vi "create_batch-default.vi"(8 "error in (no error)":errorcluster, 9 "application_command":string, 10 "application_zip":string, 11 "target_directory":path) -> (0 "error out":errorcluster, 3 "batch_file":path)   [LabVIEW 2015, in "lv-builder-l3.lvlib"]
uses:
  lv-builder-l3.lvlib
  lv-build/lv-build.lvlib
panel:
  out "batch_file":string
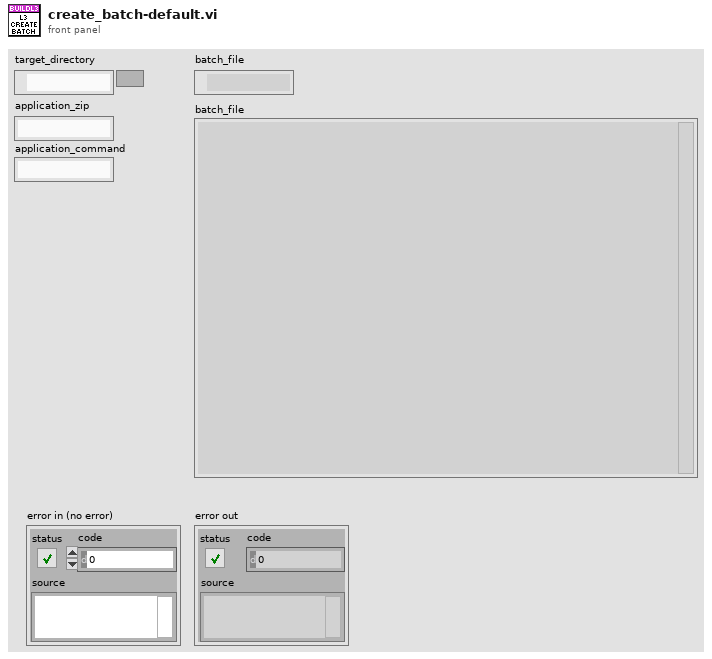
[diagram p1: front panel]
types:
  T1 = enum16{"open", "replace", "create", "open or create", "replace or create", "replace or create with confirmation"}
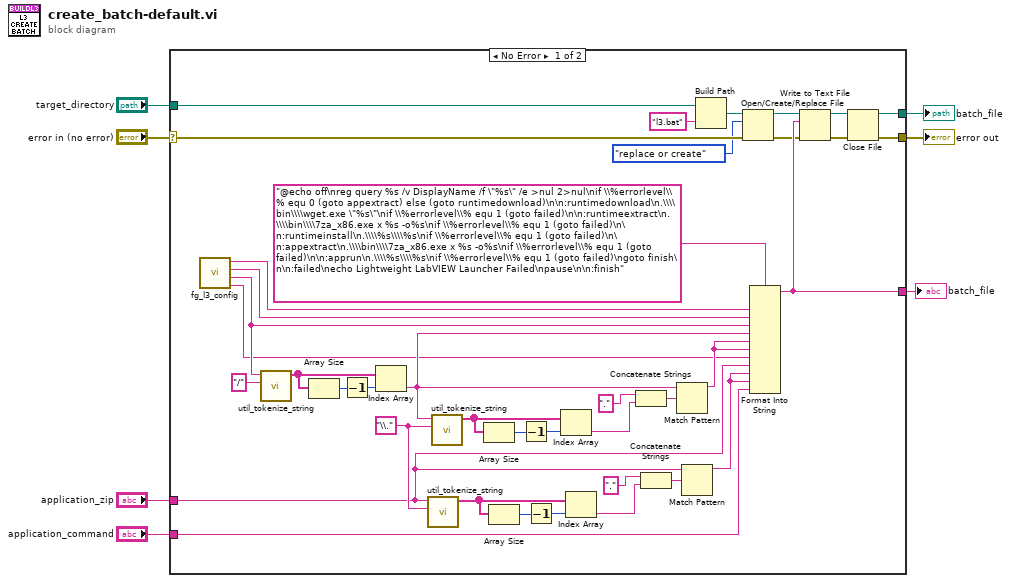
[diagram p0: block diagram]
diagram:
  n1 = case shown="No Error" "error in (no error)" {
    selector: "error in (no error)" -> [w43 w47]
    tunnel: "target_directory" -> [w9 _]
    tunnel: [w45 w47] -> w6
    tunnel: [w44 _] -> w5
    tunnel: "application_zip" -> [w16 _]
    tunnel: [w24 _] -> w2
    tunnel: "application_command" -> [w8 _]
    frame No Error {
      w26 = "\\." ("delimiter ([\\s\\t\\n\\r]+)")
      n2 = call "fg_l3_config.vi"() -> ("runtime_command"=w17:string, "runtime_address"=w20:string, "display_name"=w21:string, "registry_key"=w22:string)  [unwired: 8 in]
      n3 = call "util_tokenize_string.vi"("delimiter"="/", "input_string"=w20) -> ("delimited_string []"=w41:string[])  [unwired: 8 in, 1 out]
      n4 = Array Size(array=w41) -> (size(s)=w40:i32)
      n5 = Decrement(x=w40) -> (x-1=w39:i32)
      n6 = Index Array(array=w41, index=w39) -> (element=w19:string)
      n7 = call "util_tokenize_string.vi"("delimiter"=w26, "input_string"=w16) -> ("delimited_string []"=w27:string[])  [unwired: 8 in, 1 out]
      n8 = call "util_tokenize_string.vi"("delimiter"=w26, "input_string"=w19) -> ("delimited_string []"=w33:string[])  [unwired: 8 in, 1 out]
      n9 = Array Size(array=w33) -> (size(s)=w38:i32)
      n10 = Array Size(array=w27) -> (size(s)=w28:i32)
      n11 = Decrement(x=w38) -> (x-1=w37:i32)
      n12 = Decrement(x=w28) -> (x-1=w29:i32)
      n13 = Index Array(array=w33, index=w37) -> (element=w36:string)
      n14 = Index Array(array=w27, index=w29) -> (element=w30:string)
      n15 = Concatenate Strings("." ("string"), w36) -> (w34:string)
      n16 = Concatenate Strings("." ("string"), w30) -> (w32:string)
      n17 = Match Pattern(string=w19, regular expression=w34) -> (before substring=w18:string)  [unwired: 1 in, 3 out]
      n18 = Match Pattern(string=w16, regular expression=w32) -> (before substring=w15:string)  [unwired: 1 in, 3 out]
      n19 = Build Path(base path=w9, name or relative path="l3.bat") -> (appended path=w46:path)
      n20 = Open/Create/Replace File(file path (use dialog)=w46, error in=w43, operation (0:open)=T1."replace or create") -> (refnum out=w14:refnum<file>, error out=w11:errorcluster)  [unwired: 3 in, 1 out]
      n21 = Format Into String(format string="@echo off\nreg query %s /v DisplayName /f \"%s\" /e >nul 2>nul\nif \\%errorlevel\\% equ 0 (goto appextract) else (goto runtimedownload)\n\n:runtimedownload\n.\\\\bin\\\\wget.exe \"%s\"\nif \\%errorlevel\\% equ 1 (goto failed)\n\n:runtimeextract\n.\\\\bin\\\\7za_x86.exe x %s -o%s\nif \\%errorlevel\\% equ 1 (goto failed)\n\n:runtimeinstall\n.\\\\%s\\\\%s\nif \\%errorlevel\\% equ 1 (goto failed)\n\n:appextract\n.\\\\bin\\\\7za_x86.exe x %s -o%s\nif \\%errorlevel\\% equ 1 (goto failed)\n\n:apprun\n.\\\\%s\\\\%s\nif \\%errorlevel\\% equ 1 (goto failed)\ngoto finish\n\n:failed\necho Lightweight LabVIEW Launcher Failed\npause\n\n:finish", w22, w21, w20, w19, w18, w18, w17, w16, w15, w15, w8) -> (resulting string=w24:string)  [unwired: 2 in, 1 out]
      n22 = Write to Text File(file (use dialog)=w14, text=w24, error in=w11) -> (refnum out=w13:refnum<file>, error out=w12:errorcluster)  [unwired: 1 in, 1 out]
      n23 = Close File(refnum=w13, error in=w12) -> (path=w44:path, error out=w45:errorcluster)
    }
    frame Error {
    }
  }
  "error out" <- w6
  "batch_file" <- w5
  "batch_file" <- w2
